vi "test_CCD_Setup_Testenvironment.vi"(8 "error in":errorcluster) -> (0 "error out":errorcluster, 3 "CCD open for communication?":bool)   [LabVIEW 2023]
uses:
  Source/Classes/CCD/CCD.lvclass
  Source/Libraries/DeviceManager/DeviceManager.lvlib
panel:
  # "Connector Pane"
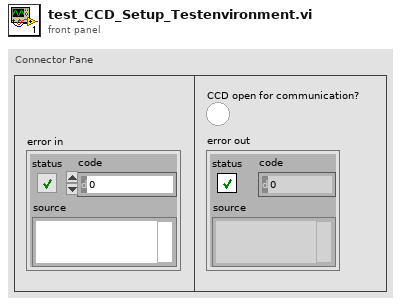
[diagram p1: front panel]
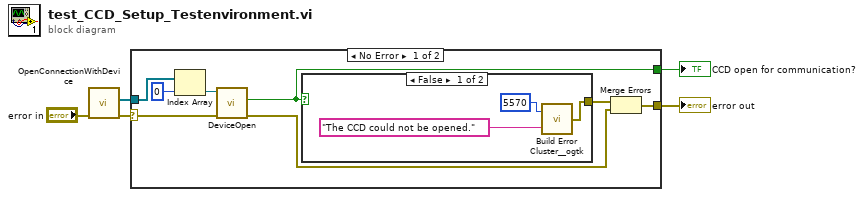
[diagram p0: block diagram]
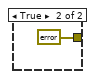
[diagram p2: hidden frame]
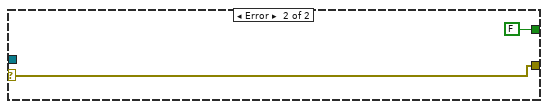
[diagram p3: hidden frame]
diagram:
  n1 = call "OpenConnectionWithDevice.vi"("error in"="error in") -> ("error out"=w4:errorcluster, "CCDs"=w5:refnum<class "CCD.lvclass">[])  [unwired: 7 in, 2 out]
  n2 = case shown="No Error" w4 {
    selector: w4 -> [w11 w19]
    tunnel: w5 -> [w13 _]
    tunnel: [w9 w19] -> w2
    tunnel: [w7 FALSE ("CCD open for communication?")] -> w1
    frame No Error {
      n3 = Index Array(array=w13, index=0) -> (element=w10:refnum<class "CCD.lvclass">)
      n4 = call-dynamic "DeviceOpen.vi"("error in (no error)"=w11, "CCD in"=w10) -> ("error out"=w6:errorcluster, "device is open?"=w7:bool)  [unwired: 6 in, 2 out]
      n5 = case shown="False" w7 {
        tunnel: [w15 errorcluster {"status"=FALSE, "code"=0, "source"=""} ("error in 2")] -> w8
        frame False {
          n6 = call <userlib>:"Build Error Cluster__ogtk.vi"("String to Prepend to source (\"\")"="The CCD could not be opened." ("String to Prepend to source (\"\")"), "code"=5570) -> ("error out"=w15:errorcluster)
        }
        frame True {
        }
      }
      n7 = Merge Errors(w8, w6) -> (w9:errorcluster)
    }
    frame Error {
    }
  }
  "error out" <- w2
  "CCD open for communication?" <- w1
